vi "Fuzzy_Input.vi"() -> ()   [LabVIEW 2016]
panel:
  in  "stop":bool
  in  "Membership Function 3":dbl[](array[numeric])
  in  "Membership Function 2":dbl[](array[numeric])
  in  "Membership Function 1":dbl[](array[numeric])
  out "XY Graph":cluster{"Array":dbl[], dbl[]}[](graph)
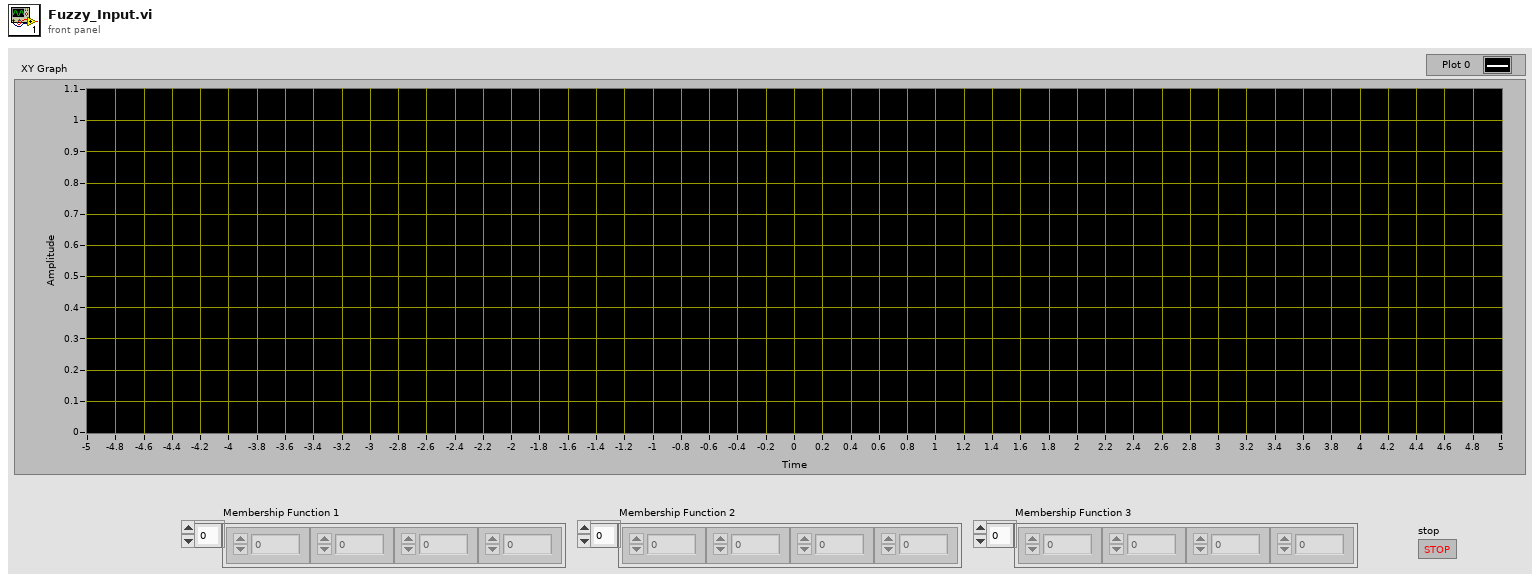
[diagram p1: front panel]
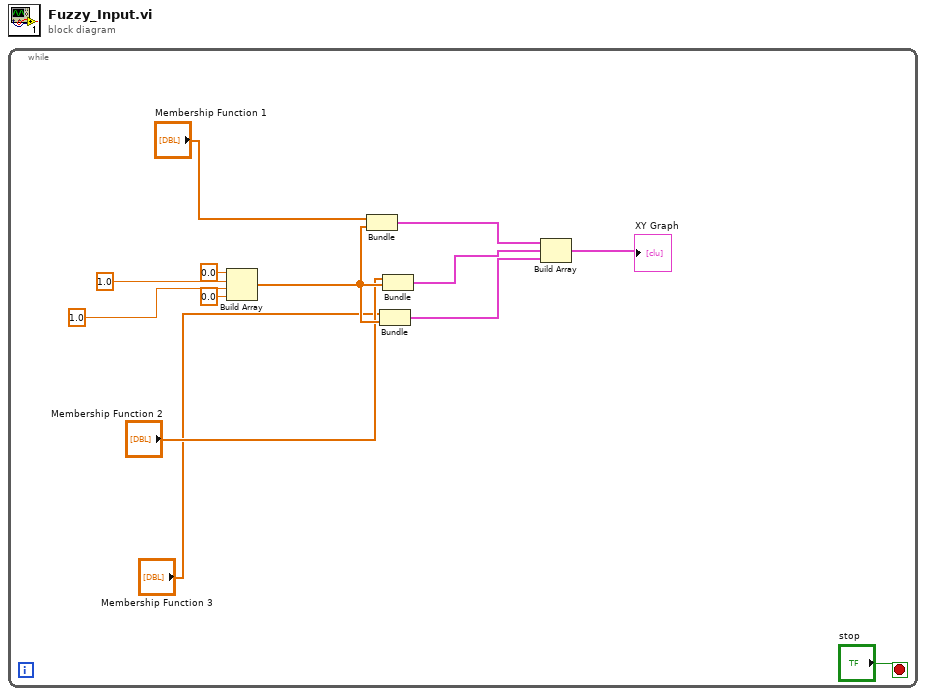
[diagram p0: block diagram]
diagram:
  n1 = while {
    stop <- "stop" stop-if-true
    n2 = Build Array(0.0 ("element"), 1.0 ("element"), 1.0 ("element"), 0.0 ("element")) -> (w5:dbl[])
    n3 = Bundle("Membership Function 1"="Membership Function 1", w5) -> (w13:cluster{"Membership Function 1":dbl[], dbl[]})  [unwired: 1 in]
    n4 = Bundle("Membership Function 3"="Membership Function 3", w5) -> (w11:cluster{"Membership Function 3":dbl[], dbl[]})  [unwired: 1 in]
    n5 = Bundle("Membership Function 2"="Membership Function 2", w5) -> (w12:cluster{"Membership Function 2":dbl[], dbl[]})  [unwired: 1 in]
    n6 = Build Array(w13, w12, w11) -> (→"XY Graph":cluster{"Membership Function 3":dbl[], dbl[]}[])
  }
